vi "Untitled 1.vi"() -> ()   [LabVIEW 2015]
uses:
  <vilib>/Utility/miscctls.llb/LVPoint32TypeDef.ctl
  <vilib>/Utility/miscctls.llb/LVPositionTypeDef.ctl
panel:
  out "reference out":refnum<vi>
  out "Position":T1
  out "Coords":T2
  in  "stop":bool
  in  "Boolean 3":bool
  in  "Boolean 2":bool
  in  "Boolean":bool
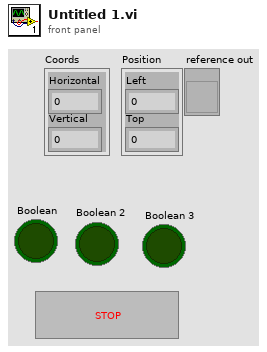
[diagram p1: front panel]
types:
  T1 = typedef "LVPositionTypeDef.ctl" = cluster{"Left":i32, "Top":i32}
  T2 = typedef "LVPoint32TypeDef.ctl" = cluster{"Horizontal":i32, "Vertical":i32}
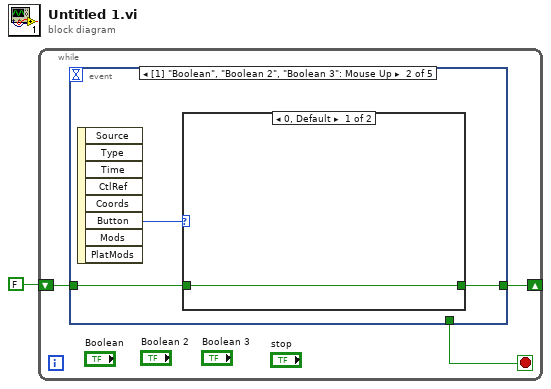
[diagram p0: block diagram]
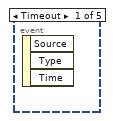
[diagram p2: hidden frame]
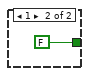
[diagram p3: hidden frame]
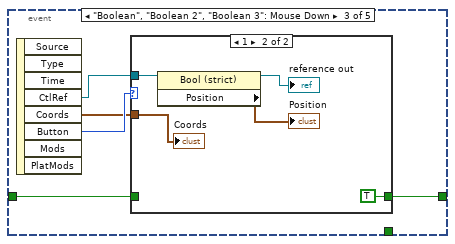
[diagram p4: hidden frame]
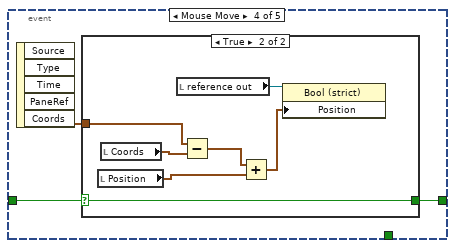
[diagram p6: hidden frame]
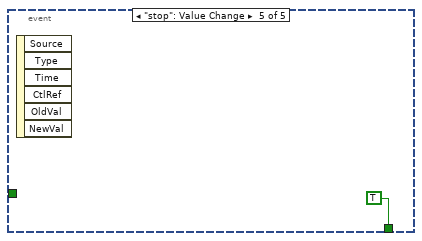
[diagram p8: hidden frame]
diagram:
  n1 = while {
    shift-right: [w3] -> _
    shift-left: FALSE -> [w4]
    stop <- w2 stop-if-true
    n2 = event shown="[1] \"Boolean\", \"Boolean 2\", \"Boolean 3\": Mouse Up" {
      selector: _ -> [_ _ _ _ _]
      dyn-events: _ -> [_ _ _ _ _]
      timeout: _ -> [_ _ _ _ _]
      tunnel: w4 -> [_ w5 w11 w22 _]
      tunnel: [_ w6 w10 w21 _] -> w3
      tunnel: [_ _ _ _ TRUE] -> w2
      event Timeout {
        n3 = event-data() -> ()  [unwired: 1 in, 3 out]
      }
      event "Boolean", "Boolean 2", "Boolean 3": Mouse Up {
        n4 = event-data() -> ("Button"=w7:u16)  [unwired: 1 in, 7 out]
        n5 = case shown="0, Default" w7 {
          tunnel: [w8 FALSE] -> w6
          tunnel: w5 -> [w8 _]
          frame 0, Default {
          }
          frame 1 {
          }
        }
      }
      event "Boolean", "Boolean 2", "Boolean 3": Mouse Down {
        n6 = event-data() -> ("CtlRef"=w13:refnum<vi>, "Coords"=w12:T2, "Button"=w14:u16)  [unwired: 1 in, 5 out]
        n7 = case shown="1" w14 {
          tunnel: w13 -> [_ w20]
          tunnel: w12 -> [_ w19]
          tunnel: w11 -> [w15 _]
          tunnel: [w15 TRUE] -> w10
          frame 0, Default {
          }
          frame 1 {
            n8 = property class="Bool (strict)"(reference=w20) -> (reference out=→"reference out":refnum<vi>, "Position"=→"Position":T1)  [unwired: 1 in, 1 out]
            "Coords" <- w19
          }
        }
      }
      event Mouse Move {
        n9 = event-data() -> ("Coords"=w23:T2)  [unwired: 1 in, 4 out]
        n10 = case shown="True" w22 {
          selector: w22 -> [w24 w25]
          tunnel: w23 -> [_ w31]
          tunnel: [w24 w25] -> w21
          frame False {
          }
          frame True {
            n11 = local read "Position"() -> (w28:T1)
            n12 = local read "Coords"() -> (w30:T2)
            n13 = local read "reference out"() -> (w27:refnum<vi>)
            n14 = Subtract(x=w31, y=w30) -> (x-y=w29:T2)
            n15 = Add(x=w29, y=w28) -> (x+y=w26:T2)
            n16 = property class="Bool (strict)"(reference=w27, "Position"=w26) -> ()  [unwired: 1 in, 2 out]
          }
        }
      }
      event "stop": Value Change {
        n17 = event-data() -> ()  [unwired: 1 in, 6 out]
      }
    }
  }
